vi "Curtin1_GetAllGroupsName.vi"(11 "Set Names in":string) -> (3 "Set Names out":string)   [LabVIEW 2022 SP3]
uses:
  <vilib>/Utility/error.llb/Trim Whitespace One-Sided.vi
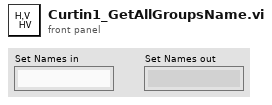
[diagram p1: front panel]
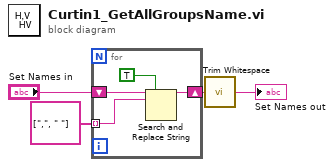
[diagram p0: block diagram]
diagram:
  n1 = for {
    shift-right: [w6] -> w4
    shift-left: "Set Names in" -> [w8]
    tunnel: string[] [",", " "] -> [w5] mode=indexing
    n2 = Search and Replace String(replace all?=TRUE ("replace all? (F)"), input string=w8, search string=w5) -> (result string=w6:string)  [unwired: 5 in, 3 out]
  }
  n3 = call <vilib>:"Trim Whitespace.vi"("string"=w4) -> ("trimmed string"=→"Set Names out":string)  [unwired: 1 in]
